vi "Find Expected Controls.vi"(8 "error in":errorcluster, 11 "vi info":T1 {"RegisterMap"."Address" format="%.0x"}) -> (0 "error out":errorcluster, 1 "Use?":bool, 2 "Controls":T8[](array[typedef]) {"Data Type" format="%.0x"}, 3 "Indicator":T8[](array[typedef]) {"Data Type" format="%.0x"}, 5 "Groups":string[](array[string]))   [LabVIEW 2019, in "Fuel Injector Analysis Addon System Explorer.lvlib"]
uses:
  Fuel Injector Analysis Addon System Explorer.lvlib
  Addon Shared/Types/Register.Info.ctl
  Addon Shared/Types/FPGA Data Types.ctl
  <vilib>/rvi/Bitfile/niFpgaBitfileStructure_VI.ctl
  <vilib>/rvi/Bitfile/nirviControlStructure.ctl
  <vilib>/rvi/Bitfile/nirviTypdefDescription.ctl
  <vilib>/rvi/Bitfile/nirviMechanicalAction.ctl
  <vilib>/rvi/Bitfile/nirviSubControlStructure.ctl
  <vilib>/rvi/Bitfile/nirviClusterElementControl.ctl
  <vilib>/picture/picture.llb/imagedata.ctl
  Support Libraries/Injection Capture IP/Types/Injection.Global.Settings.ctl
  Support Libraries/Injection Capture IP/Types/Injection.Timing.ctl
  Support Libraries/Injection Capture IP/Types/Injection.Core.Settings.ctl
  Addon Shared/Fuel Injector Analysis Addon Shared.lvlib
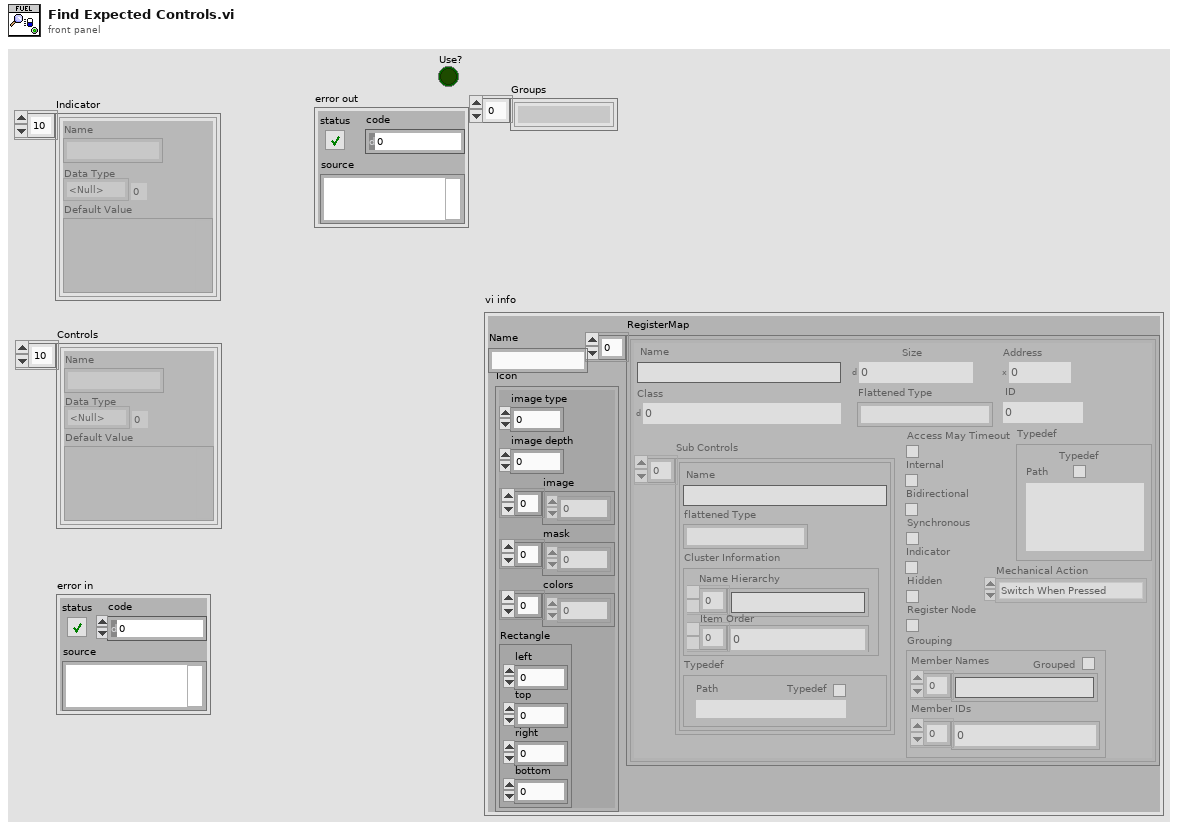
[diagram p1: front panel]
types:
  T1 = typedef "niFpgaBitfileStructure_VI.ctl" = cluster{"Name":string, "RegisterMap":T2[], "Icon":T7}
  T2 = typedef "nirviControlStructure.ctl" = cluster{"Name":string, "Hidden":bool, "Indicator":bool, "Flattened Type":string, "Grouping":cluster{"Grouped":bool, "Member Names":string[], "Member IDs":u32[]}, "Address":u32, "Size":u32, "Class":u32, "Internal":bool, "Typedef":T3, "ID":u32, "Bidirectional":bool, "Synchronous":bool, "Mechanical Action":T4, "Sub Controls":T5[], "Access May Timeout":bool, "Register Node":bool}
  T3 = typedef "nirviTypdefDescription.ctl" = cluster{"Typedef":bool, "Path":path}
  T4 = typedef "nirviMechanicalAction.ctl" = enum8{"Switch When Pressed", "Switch When Released", "Switch Until Released", "Latch When Pressed", "Latch When Released", "Latch Until Released"}
  T5 = typedef "nirviSubControlStructure.ctl" = cluster{"Name":string, "flattened Type":string, "Cluster Information":T6, "Typedef":T3}
  T6 = typedef "nirviClusterElementControl.ctl" = cluster{"Name Hierarchy":string[], "Item Order":u32[]}
  T7 = typedef "imagedata.ctl" = cluster{"image type":i32, "image depth":i32, "image":u8[], "mask":u8[], "colors":u32[], "Rectangle":cluster{"left":i16, "top":i16, "right":i16, "bottom":i16}}
  T8 = typedef "Fuel Injector Analysis Addon Shared.lvlib/Register.Info.ctl" = cluster{"Name":string, "Data Type":T9, "Default Value":variant}
  T9 = typedef "Fuel Injector Analysis Addon Shared.lvlib/FPGA Data Types.ctl" = enum8{"<Null>", "Injector.Core.Setting", "Injector.Global.Setting", "Injector.Mux.Setting", "Injector.Timing"}
  T10 = typedef "Injection.Core.Settings.ctl" = cluster{"Voltage Offset":fxp<+/-,32,8>, "Current Offset":fxp<+/-,32,8>}
  T11 = typedef "Injection.Timing.ctl" = cluster{"Injection Sample Period (Ticks)":u32}
  T12 = typedef "Injection.Global.Settings.ctl" = cluster{"Enable?":bool, "Initial Voltage Threshold":fxp<+/-,32,8>, "Event Dwell Limit":u16, "Voltage Gain":fxp<+/-,32,8>, "Current Gain":fxp<+/-,32,8>, "Filter Samples":u8, "Pretrigger Samples":u8, "Active Edge":bool}
  T13 = typedef "Type Descriptor Enumeration__ogtk.ctl" = enum8{"<Null>", "I8", "I16", "I32", "I64", "U8", "U16", "U32", "U64", "SGL", "DBL", "EXT", "CSG", "CDB", "CXT", "0x0F", "0x10", "0x11", "0x12", "0x13", "0x14", "Enum U8", "Enum U16", "Enum U32", "Enum U64", "SGL PQ", "DBL PQ", "EXT PQ", "CSG PQ", "CDB PQ", "CXT PQ", "0x1F", "0x20", "Boolean", "0x22", "0x23", "0x24", "0x25", "0x26", "0x27", "0x28", "0x29", "0x2A", "0x2B", "0x2C", "0x2D", "0x2E", "0x2F", "String", "0x31", "Path", "Pict", "0x34", "0x35", "0x36", "DAQ", "0x38", "0x39", "0x3A", "0x3B", "0x3C", "0x3D", "0x3E", "0x3F", "Array", "0x41", "0x42", "0x43", "0x44", "0x45", "0x46", "0x47", "0x48", "0x49", "0x4A", "0x4B", "0x4C", "0x4D", "0x4E", "0x4F", "Cluster", "0x51", "0x52", "Variant", "Waveform", "0x55", "0x56", "0x57", "0x58", "0x59", "0x5A", "0x5B", "0x5C", "0x5D", "0x5E", "0x5F", "0x60", "0x61", "0x62", "0x63", "0x64", "0x65", "0x66", "0x67", "0x68", "0x69", "0x6A", "0x6B", "0x6C", "0x6D", "0x6E", "0x6F", "Refnum"}
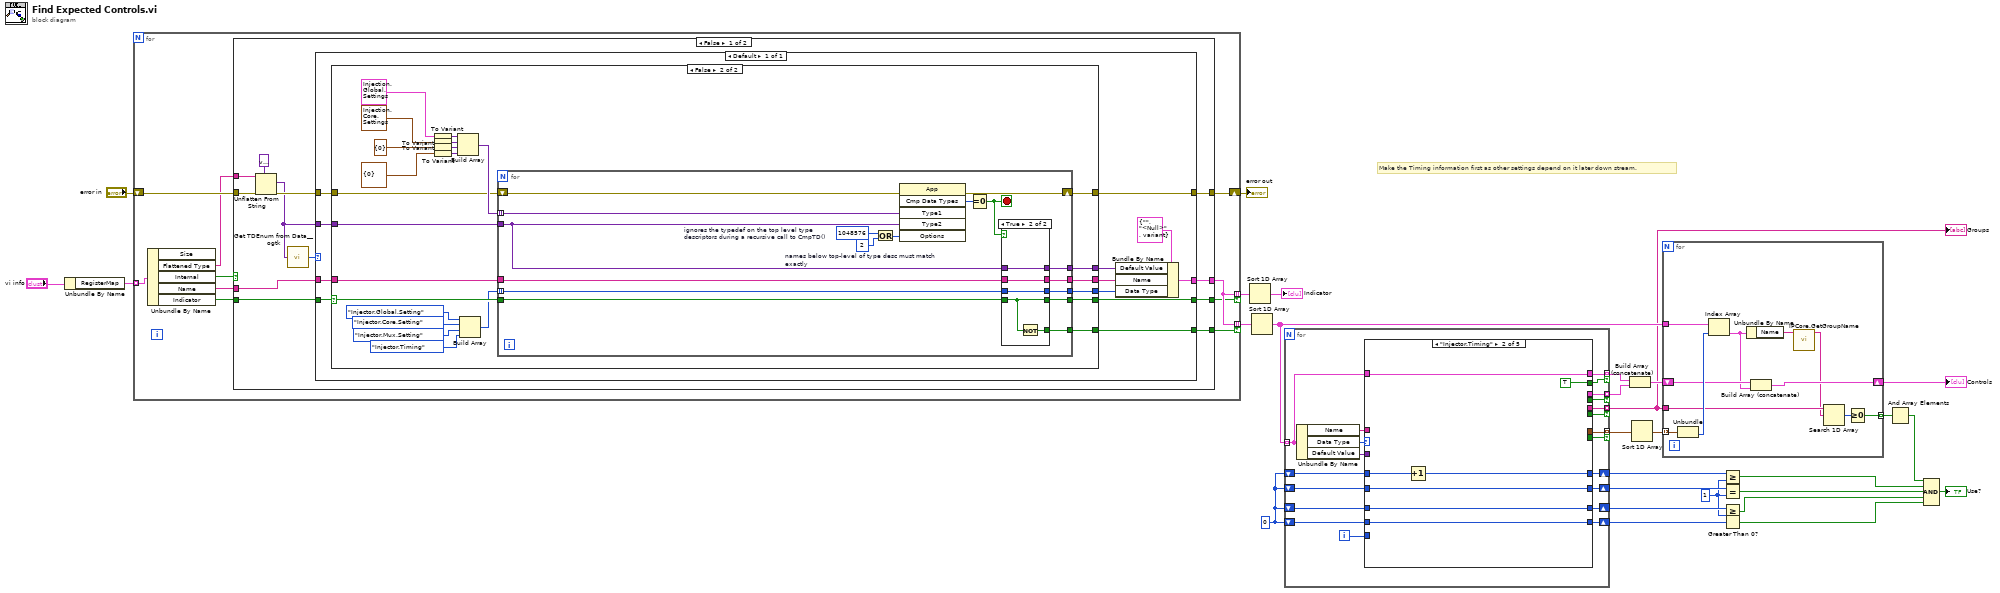
[diagram p0: block diagram]
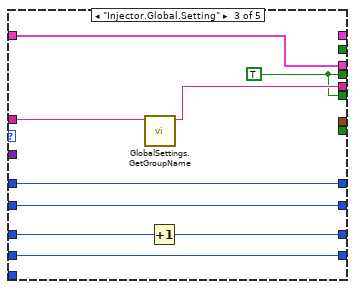
[diagram p3: hidden frame]
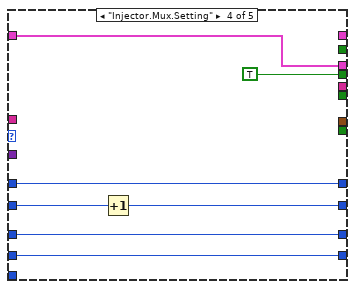
[diagram p4: hidden frame]
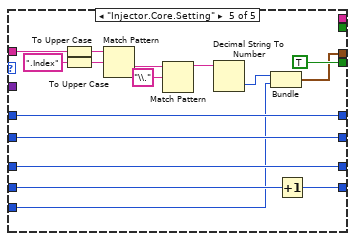
[diagram p5: hidden frame]
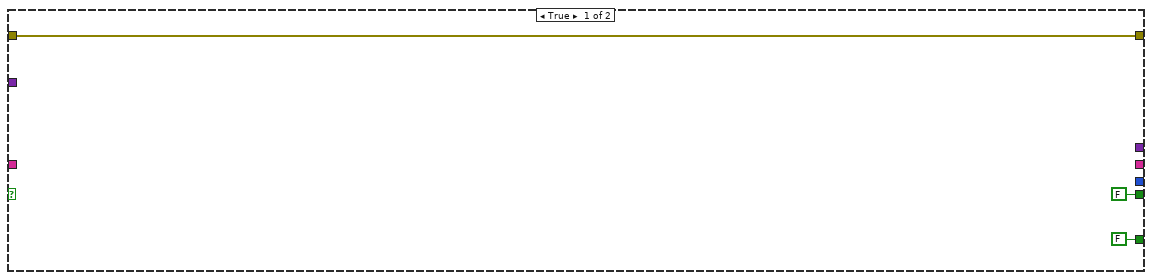
[diagram p6: hidden frame]
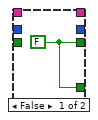
[diagram p7: hidden frame]
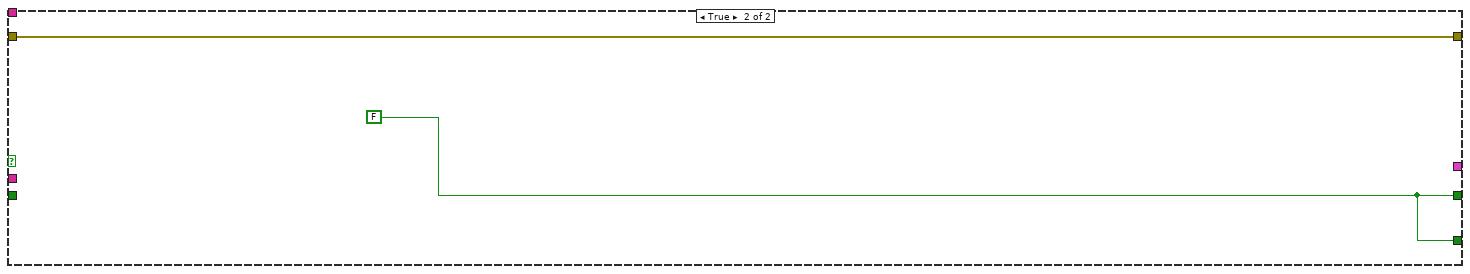
[diagram p8: hidden frame]
diagram:
  w1 = 1 ("y")
  w17 = 0
  # "Make the Timing information first as other settings depend on it later down stream."
  n1 = Unbundle By Name("vi info") -> ("RegisterMap"=w27:T2[])
  n2 = for {
    tunnel: w27 -> [w33] mode=indexing
    tunnel: [w38] -> w28 mode=indexing if=w37
    tunnel: [w38] -> w12 mode=indexing if=w36
    shift-right: [w35] -> w24
    shift-left: "error in" -> [w34]
    n3 = Unbundle By Name(w33) -> ("Flattened Type"=w29:string, "Internal"=w30:bool, "Name"=w31:string, "Indicator"=w32:bool)  [unwired: 1 out]
    n4 = case shown="False" w30 {
      tunnel: w31 -> [w49 _]
      tunnel: w32 -> [w48 _]
      tunnel: [w47 _] -> w38
      tunnel: [w46 w114] -> w37
      tunnel: [w45 w114] -> w36
      tunnel: w29 -> [w42 _]
      tunnel: [w44 w113] -> w35
      tunnel: w34 -> [w41 w113]
      frame False {
        n5 = Unflatten From String(type=variant ("Variant"), binary string=w42, error in (no error)=w41) -> (value=w39:variant, error out=w40:errorcluster)  [unwired: 3 out]
        n6 = call <userlib>:"Get TDEnum from Data__ogtk.vi"("Data"=w39) -> ("Type Descriptor Enumeration"=w50:T13)  [unwired: 4 in]
        n7 = case shown="Default" w50 {
          tunnel: [w62] -> w46
          tunnel: w48 -> [w57]
          tunnel: w49 -> [w58]
          tunnel: [w59] -> w47
          tunnel: [w61] -> w45
          tunnel: w39 -> [w56]
          tunnel: [w52] -> w44
          tunnel: w40 -> [w51]
          frame Default {
            n8 = case shown="False" w57 {
              selector: w57 -> [_ w86]
              tunnel: [FALSE ("Boolean") w89] -> w62
              tunnel: [FALSE ("Boolean") w88] -> w61
              tunnel: w58 -> [_ w87]
              tunnel: w56 -> [_ w82]
              tunnel: [_ w81] -> w55
              tunnel: [_ w80] -> w54
              tunnel: [_ w79] -> w53
              tunnel: [w65 w74] -> w52
              tunnel: w51 -> [w65 w75]
              frame True {
              }
              frame False {
                n9 = To Variant(anything=T12 {"Enable?"=FALSE, "Initial Voltage Threshold"=0.0, "Event Dwell Limit"=0, "Voltage Gain"=0.0, "Current Gain"=1.0, "Filter Samples"=5, "Pretrigger Samples"=5, "Active Edge"=TRUE} ("InjectorAnalysis.Settings")) -> (Variant=w85:variant)
                n10 = To Variant(anything=T10 {"Voltage Offset"=0.0, "Current Offset"=0.0} ("Index<#>.<UserName>")) -> (Variant=w77:variant)
                n11 = To Variant(anything=cluster{"# of Injectors":u8} {"# of Injectors"=0} ("Injector.MUX.Settings")) -> (Variant=w76:variant)
                n12 = To Variant(anything=T11 {"Injection Sample Period (Ticks)"=0} ("Injector.Timing")) -> (Variant=w73:variant)
                n13 = Build Array(w85, w77, w76, w73) -> (w83:variant[])
                n14 = Build Array(FPGA_Data_Types."Injector.Global.Setting" ("Data Type"), FPGA_Data_Types."Injector.Core.Setting" ("Data Type"), FPGA_Data_Types."Injector.Mux.Setting" ("Data Type"), FPGA_Data_Types."Injector.Timing" ("Data Type")) -> (w78:T9[])
                n15 = for {
                  tunnel: w82 -> [w95]
                  tunnel: [w104] -> w88
                  tunnel: w87 -> [w103]
                  tunnel: w83 -> [w94] mode=indexing
                  tunnel: [w102] -> w80
                  tunnel: [w101] -> w81
                  tunnel: [w100] -> w79
                  tunnel: w78 -> [w99] mode=indexing
                  tunnel: w86 -> [w106]
                  tunnel: [w105] -> w89
                  shift-right: [w90] -> w74
                  shift-left: w75 -> [w91]
                  stop <- w92 stop-if-true
                  w97 = 2  # names below top-level of type desc must match exactly
                  w96 = 1048576  # ignores the typedef on the top level type descriptors during a recursive call to CmpTD()
                  n16 = Or(x=w96, y=w97) -> (x .or. y?=w98:i32)
                  n17 = invoke class="App" method="Cmp Data Types"(error in=w91, "Type1"=w94, "Type2"=w95, "Options"=w98) -> (error out=w90:errorcluster, "Compare Data Types"=w93:i32)  [unwired: 2 in, 4 out]
                  n18 = Equal To 0?(x=w93) -> (x = 0?=w92:bool)
                  n19 = case shown="True" w92 {
                    tunnel: w106 -> [_ w112]
                    tunnel: [w107 w112] -> w105
                    tunnel: [w107 w111] -> w104
                    tunnel: w103 -> [_ w109]
                    tunnel: [_ w110] -> w102
                    tunnel: w95 -> [_ w110]
                    tunnel: [_ w109] -> w101
                    tunnel: [_ w108] -> w100
                    tunnel: w99 -> [_ w108]
                    frame False {
                      w107 = FALSE ("Boolean")
                    }
                    frame True {
                      n20 = Not(x=w112) -> (.not. x?=w111:bool)
                    }
                  }
                }
              }
            }
            n21 = Bundle By Name(cluster=T8 {"Name"="", "Data Type"=enum."<Null>", "Default Value"=variant(refnum<class> refnum)}, "Default Value"=w54, "Name"=w55, "Data Type"=w53) -> (w59:T8)
          }
        }
      }
      frame True {
        w114 = FALSE ("Boolean")
      }
    }
  }
  "error out" <- w24
  n22 = Sort 1D Array(array=w28) -> (sorted array=→"Indicator":T8[])
  n23 = Sort 1D Array(array=w12) -> (sorted array=w10:T8[])
  n24 = for {
    tunnel: w10 -> [w121] mode=indexing
    shift-right: [w133] -> w16
    shift-left: w17 -> [w134]
    shift-right: [w132] -> w21
    shift-left: w17 -> [w131]
    shift-right: [w129] -> w15
    shift-left: w17 -> [w128]
    shift-right: [w126] -> w22
    shift-left: w17 -> [w127]
    tunnel: [w124] -> w11 mode=indexing if=w123
    tunnel: [w120] -> w7 mode=indexing if=w119
    tunnel: [w118] -> w6 mode=indexing if=w116
    tunnel: [w117] -> w4 mode=indexing if=w115
    i -> [w122]
    n25 = Unbundle By Name(w121) -> ("Name"=w125:string, "Data Type"=w135:T9, "Default Value"=w130:variant)
    n26 = case shown="\"Injector.Timing\"" w135 {
      tunnel: w134 -> [w139 w146 w155 w162 w178]
      tunnel: [w139 w146 w155 w162 w177] -> w133
      tunnel: [w138 w145 w153 w161 w176] -> w132
      tunnel: w131 -> [w138 w145 w154 w161 w176]
      tunnel: w130 -> [_ _ _ _ _]
      tunnel: [w137 w144 w152 w158 w175] -> w129
      tunnel: w128 -> [w137 w144 w152 w159 w175]
      tunnel: w127 -> [w136 w143 w151 w160 w174]
      tunnel: [w136 w142 w151 w160 w174] -> w126
      tunnel: [_ _ _ _ TRUE] -> w123
      tunnel: w125 -> [_ _ w149 _ w172]
      tunnel: [_ _ _ _ w164] -> w124
      tunnel: w122 -> [_ _ _ _ w163]
      tunnel: w121 -> [_ w141 w150 w157 _]
      tunnel: [_ w141 _ _ _] -> w120
      tunnel: [_ TRUE _ _ _] -> w119
      tunnel: [_ _ w150 w157 _] -> w118
      tunnel: [_ _ w147 TRUE _] -> w116
      tunnel: [_ _ w148 _ _] -> w117
      tunnel: [_ _ w147 _ _] -> w115
      frame "<Null>", Default {
      }
      frame "Injector.Timing" {
        n27 = Increment(x=w143) -> (x+1=w142:i32)
      }
      frame "Injector.Global.Setting" {
        w147 = TRUE
        n28 = call "GlobalSettings.GetGroupName.vi"("Name"=w149) -> ("Group"=w148:string)  [unwired: 10 in]
        n29 = Increment(x=w154) -> (x+1=w153:i32)
      }
      frame "Injector.Mux.Setting" {
        n30 = Increment(x=w159) -> (x+1=w158:i32)
      }
      frame "Injector.Core.Setting" {
        n31 = To Upper Case(1:w172) -> (0:w170:string)
        n32 = To Upper Case(1:".Index" ("regular expression")) -> (0:w169:string)
        n33 = Match Pattern(string=w170, regular expression=w169) -> (after substring=w168:string)  [unwired: 1 in, 3 out]
        n34 = Match Pattern(string=w168, regular expression="\\.") -> (before substring=w166:string)  [unwired: 1 in, 3 out]
        n35 = Decimal String To Number(string=w166) -> (number=w165:i32)  [unwired: 2 in, 1 out]
        n36 = Bundle(w165, w163) -> (w164:cluster{i32, i32})  [unwired: 1 in]
        n37 = Increment(x=w178) -> (x+1=w177:i32)
      }
    }
  }
  "Groups" <- w4
  n38 = Build Array (concatenate)(w7, w6) -> (w5:T8[])
  n39 = Sort 1D Array(array=w11) -> (sorted array=w9:cluster{i32, i32}[])
  n40 = for {
    shift-right: [w185] -> w8
    shift-left: w5 -> [w186]
    tunnel: w10 -> [w189]
    tunnel: w9 -> [w188] mode=indexing
    tunnel: w4 -> [w182]
    tunnel: [w179] -> w3 mode=indexing
    n41 = Unbundle(w188) -> (w187:i32)  [unwired: 1 out]
    n42 = Index Array(array=w189, index=w187) -> (element=w184:T8)
    n43 = Unbundle By Name(w184) -> ("Name"=w183:string)
    n44 = Build Array (concatenate)(w186, w184) -> (w185:T8[])
    n45 = call "IPCore.GetGroupName.vi"("Name"=w183) -> ("Group"=w181:string)  [unwired: 10 in]
    n46 = Search 1D Array(1D array=w182, element=w181) -> (index of element=w180:i32)  [unwired: 1 in]
    n47 = Greater Or Equal To 0?(x=w180) -> (x >= 0?=w179:bool)
  }
  "Controls" <- w8
  n48 = Greater Or Equal?(x=w22, y=w1) -> (x >= y?=w19:bool)
  n49 = Equal?(x=w15, y=w1) -> (x = y?=w13:bool)
  n50 = Greater Or Equal?(x=w21, y=w1) -> (x >= y?=w14:bool)
  n51 = Greater Than 0?(x=w16) -> (x > 0?=w20:bool)
  n52 = And Array Elements(Boolean array=w3) -> (logical AND=w2:bool)
  n53 = Compound Arithmetic op=AND(w2, w19, w13, w14, w20) -> (→"Use?":bool)
